vi "Configure_Voltage.vi"(8 "error in (no error)":errorcluster, 10 "DC_Voltage_Configuration":variant, 11 "NI-DMM in":refnum<class "NI-DMM.lvclass">) -> (0 "error out":errorcluster, 3 "NI-DMM out":refnum<class "NI-DMM.lvclass">)   [LabVIEW 2020, in "NI-DMM.lvclass"]
uses:
  NI-DMM.lvclass
  C:/Program Files/National Instruments/LabVIEW 2020/vi.lib/MeasurementLink/MeasurementLink Instrument/ISession Factory/ISession Factory.lvclass
  Typedefs/Configure_Parameters.ctl
  <vilib>/MeasurementLink/MeasurementLink Session Management V1/Session Reservation/Pin Type.ctl
  Typedefs/connection with session.ctl
  <vilib>/MeasurementLink/MeasurementLink Session Management V1/Session Reservation/Connection.ctl
  <instrlib>/niDMM/nidmm.llb/niDMM Resolution in Digits.ctl
  f01df658-2e31-4a97-abfd-bc2b634ba6ad.vi
  <vilib>/MeasurementLink/MeasurementLink Session Management V1/Session Reservation/Get Connections Impl.vi
  <instrlib>/niDMM/nidmm.llb/niDMM Configure Measurement Digits.vi
  <vilib>/MeasurementLink/MeasurementLink Session Management V1/Session Reservation/Session Reservation.lvclass
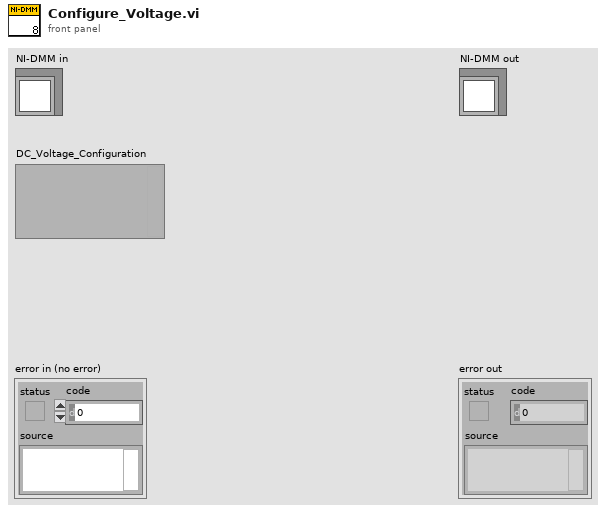
[diagram p1: front panel]
types:
  T1 = typedef "NI-DMM.lvclass/connection with session.ctl" = cluster{"session":refnum<k15>, "connection":T2}
  T2 = typedef "MeasurementLink Session Management V1.lvlib/Session Reservation.lvclass/Connection.ctl" = cluster{"pin or relay name":string, "site":i32, "instrument type id":string, "channel":string}
  T3 = typedef "MeasurementLink Session Management V1.lvlib/Session Reservation.lvclass/Pin Type.ctl" = enum16{"DUT and System Pins", "System Pins"}
  T4 = typedef "NI-DMM.lvclass/Configure_Parameters.ctl" = cluster{"pin name":string[], "Range":dbl, "Measurement Type":enum32{"DC Volts", "AC Volts", "DC Current", "AC Current", "2-wire Resistance", "4-wire Resistance", "Diode", "Frequency", "Period", "AC Volts DC Coupled", "Capacitance", "Inductance", "Temperature"}, "Resolution in Digits":enum32{"3 1/2", "4 1/2", "5 1/2", "6 1/2", "7 1/2"}}
  T5 = enum32{"3 1/2", "4 1/2", "5 1/2", "6 1/2", "7 1/2"}
  T6 = enum32{"DC Volts", "AC Volts", "DC Current", "AC Current", "2-wire Resistance", "4-wire Resistance", "Diode", "Frequency", "Period", "AC Volts DC Coupled", "Capacitance", "Inductance", "Temperature"}
  T7 = typedef "niDMM Resolution in Digits.ctl" = dbl
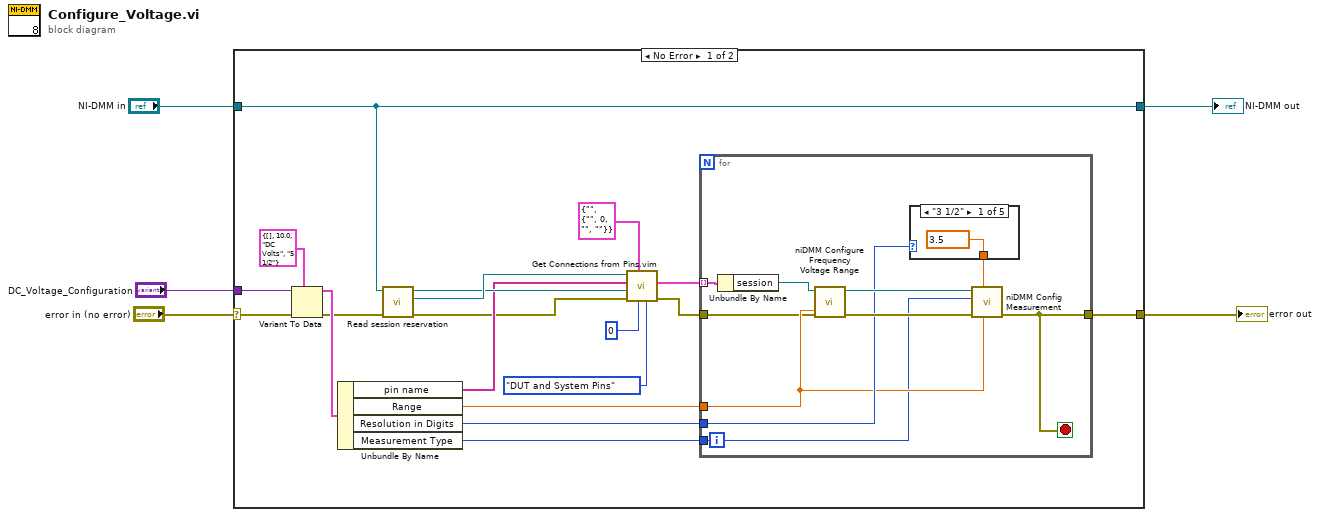
[diagram p0: block diagram]
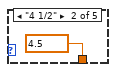
[diagram p2: hidden frame]
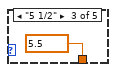
[diagram p3: hidden frame]
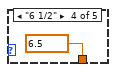
[diagram p4: hidden frame]
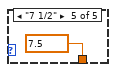
[diagram p5: hidden frame]
diagram:
  n1 = case shown="No Error" "error in (no error)" {
    selector: "error in (no error)" -> [w24 w40]
    tunnel: "DC_Voltage_Configuration" -> [w23 _]
    tunnel: [w18 w40] -> w3
    tunnel: "NI-DMM in" -> [w13 w41]
    tunnel: [w13 w41] -> w1
    frame No Error {
      n2 = Variant To Data(error in=w24, type=T4 {"pin name"=[], "Range"=10.0, "Measurement Type"=enum."DC Volts", "Resolution in Digits"=enum."5 1/2"}, Variant=w23) -> (data=w21:T4, error out=w16:errorcluster)
      n3 = Unbundle By Name(w21) -> ("pin name"=w10:string[], "Range"=w19:dbl, "Resolution in Digits"=w20:T5, "Measurement Type"=w17:T6)
      n4 = call-dynamic "Read session reservation.vi"("error in (no error)"=w16, "Abstract_Instrument in"=w13) -> ("error out"=w7:errorcluster, "Session Reservation.lvclass"=w12:refnum<class "Session Reservation.lvclass">, "Abstract_Instrument out"=w11:refnum<class "NI-DMM.lvclass">)  [unwired: 7 in]
      n5 = call "Get Connections from Pins.vim"("pin type"=Pin_Type."DUT and System Pins", "site"=0, "connection type"=T1 {"session"="", "connection"={"pin or relay name"="", "site"=0, "instrument type id"="", "channel"=""}}, "error in"=w7, "session factory"=w11, "pin or relay names"=w10, "session reservation in"=w12) -> ("error out"=w6:errorcluster, "connections"=w8:T1[])  [unwired: 2 in, 1 out]
      n6 = for {
        tunnel: w20 -> [w31]
        tunnel: w19 -> [w30]
        tunnel: [w25] -> w18
        tunnel: w17 -> [w29]
        tunnel: w8 -> [w28] mode=indexing
        tunnel: w6 -> [w26]
        stop <- w25 stop-if-true
        n7 = Unbundle By Name(w28) -> ("session"=w27:refnum<k15>)
        n8 = call <instrlib>:"niDMM Configure Frequency Voltage Range.vi"("Frequency Voltage Range"=w30, "error in (no error)"=w26, "instrument handle"=w27) -> ("error out"=w32:errorcluster, "instrument handle out"=w33:refnum<k15>)  [unwired: 7 in]
        n9 = case shown="\"3 1/2\"" w31 {
          tunnel: [w35 w36 w37 w38 w39] -> w34
          frame "3 1/2" {
            w35 = T7 3.5 items=["3 1/2"=3.5, "4 1/2"=4.5, "5 1/2"=5.5, "6 1/2"=6.5, "7 1/2"=7.5] ("Resolution in Digits")
          }
          frame "4 1/2" {
            w36 = T7 4.5 items=["3 1/2"=3.5, "4 1/2"=4.5, "5 1/2"=5.5, "6 1/2"=6.5, "7 1/2"=7.5] ("Resolution in Digits")
          }
          frame "5 1/2" {
            w37 = T7 5.5 items=["3 1/2"=3.5, "4 1/2"=4.5, "5 1/2"=5.5, "6 1/2"=6.5, "7 1/2"=7.5] ("Resolution in Digits")
          }
          frame "6 1/2" {
            w38 = T7 6.5 items=["3 1/2"=3.5, "4 1/2"=4.5, "5 1/2"=5.5, "6 1/2"=6.5, "7 1/2"=7.5] ("Resolution in Digits")
          }
          frame "7 1/2" {
            w39 = T7 7.5 items=["3 1/2"=3.5, "4 1/2"=4.5, "5 1/2"=5.5, "6 1/2"=6.5, "7 1/2"=7.5] ("Resolution in Digits")
          }
        }
        n10 = call-poly <instrlib>:"niDMM Config Measurement.vi"("Range"=w30, "Resolution in Digits"=w34, "error in (no error)"=w32, "Function"=w29, "instrument handle"=w33) -> ("error out"=w25:errorcluster)  [unwired: 5 in, 1 out]
      }
    }
    frame Error {
    }
  }
  "error out" <- w3
  "NI-DMM out" <- w1
